vi "P4CMDSub Check for P4V.vi"(8 "error in (no error)":errorcluster) -> (0 "error out":errorcluster, 2 "visual client path":string, 5 "visual client found?":bool)   [LabVIEW 2017, in "NI_SCC_P4CMD.lvlib"]
uses:
  <vilib>/SourceControl/Providers/P4CMD/NI_SCC_P4CMD.lvlib
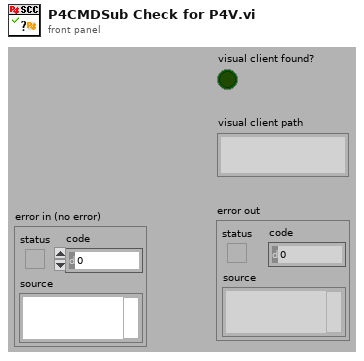
[diagram p1: front panel]
types:
  T1 = enum32{"invalid OS target", "Mac OS", "Windows 3.1", "Windows 95/NT", "Solaris 1", "Solaris 2", "HP-UX", "PowerMAX", "Linux", "Irix", "Rhapsody", "BeOS", "AIX", "OSF1", "VxWorks", "PharLap", "Carbon", "RTX", "Windows x64", "Linux x64", "Mac OS X x64"}
  T2 = enum32{"KEY_QUERY_VALUE", "KEY_SET_VALUE", "KEY_CREATE_SUB_KEY", "KEY_ENUMERATE_SUB_KEYS", "KEY_NOTIFY", "KEY_CREATE_LINK", "KEY_READ", "KEY_WRITE", "KEY_ALL_ACCESS", "KEY_READ | KEY_WRITE"}
  T3 = enum32{"HKEY_CLASSES_ROOT", "HKEY_CURRENT_USER", "HKEY_LOCAL_MACHINE", "HKEY_USERS", "HKEY_PERFORMANCE_DATA", "HKEY_CURRENT_CONFIG", "HKEY_DYN_DATA"}
  T4 = typedef "Registry refnum.ctl" = refnum<k1>
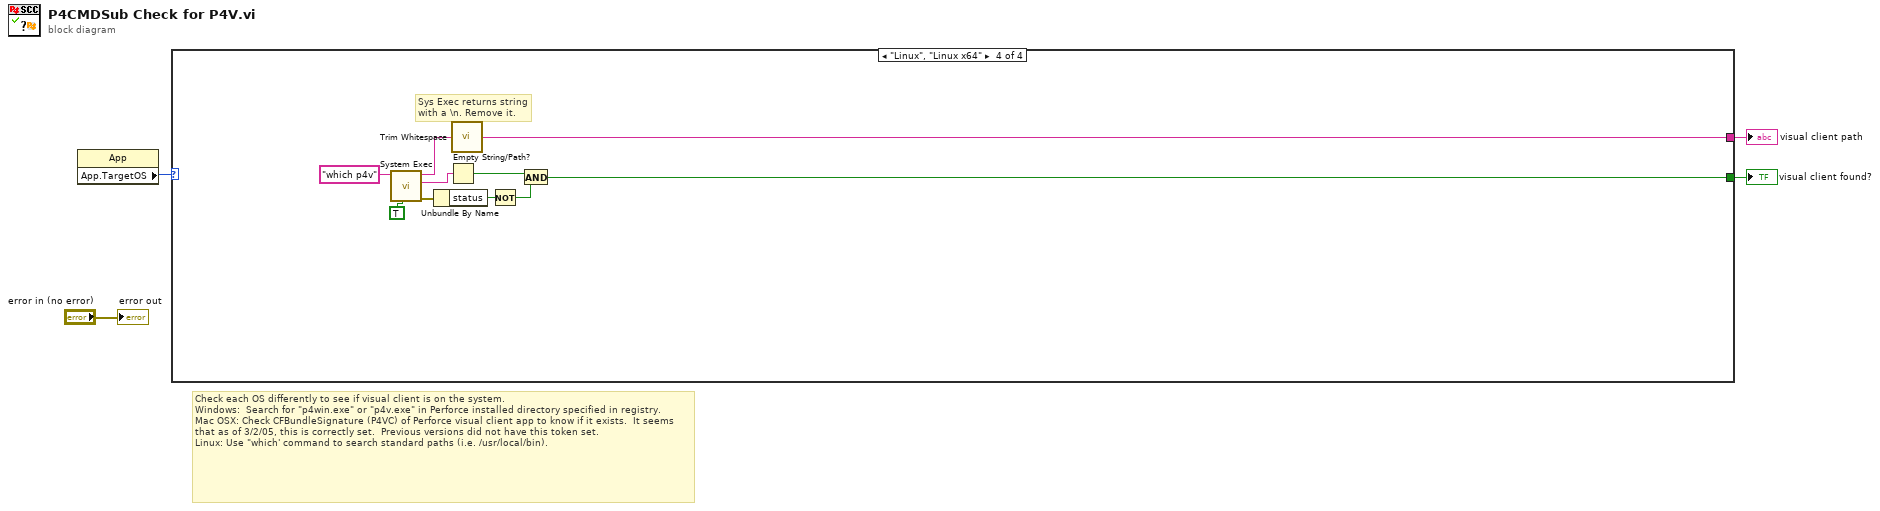
[diagram p0: block diagram]
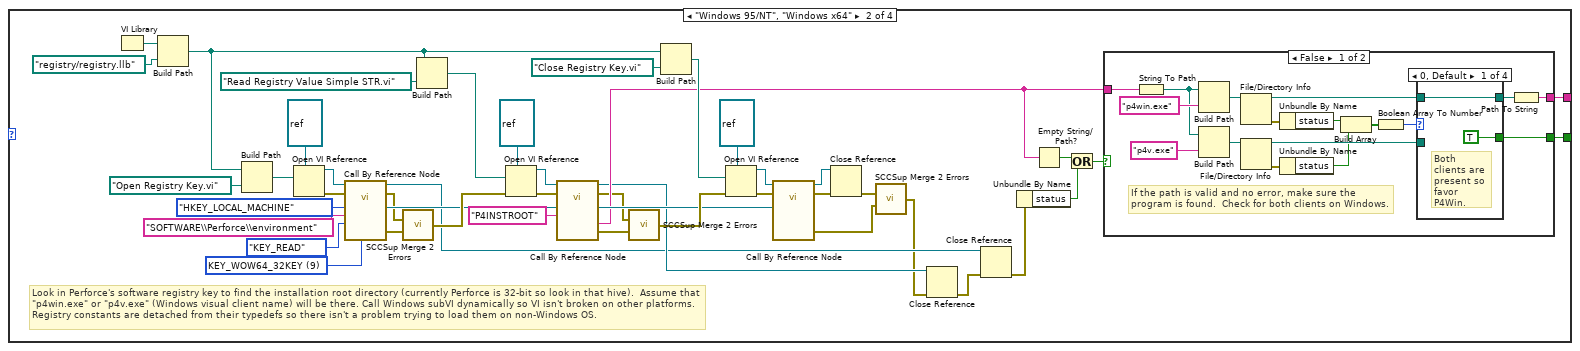
[diagram p3: hidden frame]
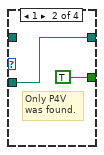
[diagram p4: hidden frame]
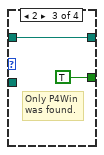
[diagram p5: hidden frame]
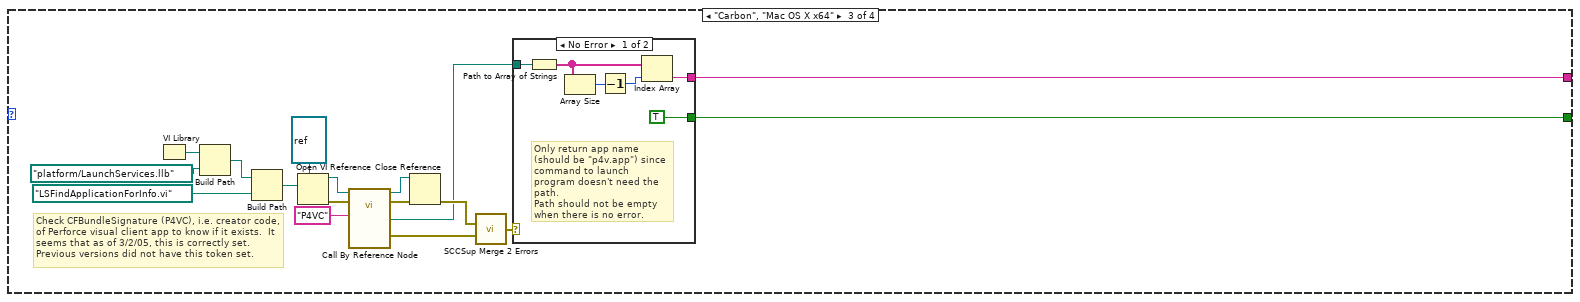
[diagram p8: hidden frame]
diagram:
  # "Check each OS differently to see if visual client is on the system. \nWindows:  Search for \"p4win.exe\" or \"p4v.exe\" in Perforce installed directory specified in registry.\nMac OSX: Check CFBundleSignature (P4VC) of Perforce visual client app to know if it exists.  It seems that as of 3/2/05, this is correctly set.  Previous versions did not have this token set.\nLinux: Use \"which' command to search standard paths (i.e. /usr/local/bin)."
  n1 = property on="Property Node" class="App"() -> ("App.TargetOS"=w3:T1)  [unwired: 2 in, 2 out]
  n2 = case shown="\"Linux\", \"Linux x64\"" w3 {
    tunnel: [_ w41 w90 w98] -> w2
    tunnel: [_ w42 w89 w97] -> w1
    frame Default {
      # "For all OS's not supporting, assume not found."
    }
    frame "Windows 95/NT", "Windows x64" {
      w5 = u16 9 items=["Default"=0, "KEY_WOW64_64KEY"=8, "KEY_WOW64_32KEY"=9] ("registry view")
      # "Look in Perforce's software registry key to find the installation root directory (currently Perforce is 32-bit so look in that hive).  Assume that \"p4win.exe\" or \"p4v.exe\" (Windows visual client name) will be there. Call Windows subVI dynamically so VI isn't broken on other platforms.  \nRegistry constants are detached from their typedefs so there isn't a problem trying to load them on non-Windows OS."
      n3 = VI Library() -> (path=w14:path)
      n4 = Build Path(base path=w14, name or relative path=path "registry/registry.llb" ("stripped path")) -> (appended path=w17:path)
      n5 = Build Path(base path=w17, name or relative path=path "Open Registry Key.vi" ("stripped path")) -> (appended path=w45:path)
      n6 = Open VI Reference(type specifier VI Refnum (for type only)=refnum<vi> refnum, vi path=w45) -> (vi reference=w47:refnum<vi>, error out=w46:errorcluster)  [unwired: 1 in, 3 out]
      n7 = call-by-ref "Call By Reference Node"(reference=w47, error in=w46, "registry view"=w5, "security access mask (KEY_READ | KEY_WRITE)"=T2."KEY_READ", "subkey"="SOFTWARE\\Perforce\\environment", "root key (HKEY_LOCAL_MACHINE)"=T3."HKEY_LOCAL_MACHINE") -> (reference out=w8:refnum<vi>, error out=w12:errorcluster, 0:"error out"=w44:errorcluster, "refnum out"=w16:T4)  [unwired: 6 in]
      n8 = call <vilib>:"SCCSup Merge 2 Errors.vi"("Error IO 1"=w12, "Error IO 2"=w44) -> ("Error IO out"=w24:errorcluster)  [unwired: 13 out]
      n9 = Build Path(base path=w17, name or relative path=path "Read Registry Value Simple STR.vi" ("stripped path")) -> (appended path=w20:path)
      n10 = Open VI Reference(type specifier VI Refnum (for type only)=refnum<vi> refnum, vi path=w20, error in (no error)=w24) -> (vi reference=w33:refnum<vi>, error out=w34:errorcluster)  [unwired: 3 out]
      n11 = call-by-ref "Call By Reference Node"(reference=w33, error in=w34, "value"="P4INSTROOT" ("subkey"), "refnum"=w16) -> (reference out=w10:refnum<vi>, error out=w11:errorcluster, 0:"error out"=w35:errorcluster, "String/Binary data"=w13:string, "refnum out"=w15:T4)  [unwired: 4 in, 1 out]
      n12 = call <vilib>:"SCCSup Merge 2 Errors.vi"("Error IO 1"=w11, "Error IO 2"=w35) -> ("Error IO out"=w21:errorcluster)  [unwired: 13 out]
      n13 = Build Path(base path=w17, name or relative path=path "Close Registry Key.vi" ("stripped path")) -> (appended path=w19:path)
      n14 = Open VI Reference(type specifier VI Refnum (for type only)=refnum<vi> refnum, vi path=w19, error in (no error)=w21) -> (vi reference=w28:refnum<vi>, error out=w27:errorcluster)  [unwired: 3 out]
      n15 = call-by-ref "Call By Reference Node"(reference=w28, error in=w27, "refnum"=w15) -> (reference out=w31:refnum<vi>, error out=w30:errorcluster, 0:"error out"=w26:errorcluster)  [unwired: 6 in]
      n16 = Close Reference(reference=w31, error in (no error)=w30) -> (error out=w25:errorcluster)
      n17 = call <vilib>:"SCCSup Merge 2 Errors.vi"("Error IO 1"=w25, "Error IO 2"=w26) -> ("Error IO out"=w7:errorcluster)  [unwired: 13 out]
      n18 = Close Reference(reference=w10, error in (no error)=w7) -> (error out=w9:errorcluster)
      n19 = Close Reference(reference=w8, error in (no error)=w9) -> (error out=w6:errorcluster)
      n20 = Unbundle By Name(w6) -> ("status"=w50:bool)
      n21 = Empty String/Path?(string/path=w13) -> (empty?=w49:bool)
      n22 = Or(x=w49, y=w50) -> (x .or. y?=w43:bool)
      n23 = case shown="False" w43 {
        tunnel: [w59 _] -> w42
        tunnel: [w67 _] -> w41
        tunnel: w13 -> [w65 _]
        frame False {
          # "If the path is valid and no error, make sure the program is found.  Check for both clients on Windows."
          n24 = String To Path(string=w65) -> (path=w62:path)
          n25 = Build Path(base path=w62, name or relative path="p4win.exe" ("subkey")) -> (appended path=w64:path)
          n26 = Build Path(base path=w62, name or relative path="p4v.exe" ("subkey")) -> (appended path=w58:path)
          n27 = File/Directory Info(path=w64) -> (path out=w61:path, error out=w57:errorcluster)  [unwired: 1 in, 5 out]
          n28 = File/Directory Info(path=w58) -> (path out=w55:path, error out=w56:errorcluster)  [unwired: 1 in, 5 out]
          n29 = Unbundle By Name(w57) -> ("status"=w54:bool)
          n30 = Unbundle By Name(w56) -> ("status"=w53:bool)
          n31 = Build Array(w54, w53) -> (w52:bool[])
          n32 = Boolean Array To Number(Boolean array=w52) -> (number=w51:u32)
          n33 = case shown="0, Default" w51 {
            tunnel: w61 -> [w68 _ w72 _]
            tunnel: [w68 w70 w72 _] -> w60
            tunnel: [TRUE TRUE TRUE _] -> w67
            tunnel: w55 -> [_ w70 _ _]
            frame 0, Default {
              # "Both clients are present so favor P4Win."
            }
            frame 1 {
              # "Only P4V was found."
            }
            frame 2 {
              # "Only P4Win was found."
            }
            frame 3 {
              # "Neither clients were found."
            }
          }
          n34 = Path To String(path=w60) -> (string=w59:string)
        }
        frame True {
          # "Path is empty or an error occurred so say client was not found."
        }
      }
    }
    frame "Carbon", "Mac OS X x64" {
      # "Check CFBundleSignature (P4VC), i.e. creator code, of Perforce visual client app to know if it exists.  It seems that as of 3/2/05, this is correctly set.  Previous versions did not have this token set."
      n35 = VI Library() -> (path=w85:path)
      n36 = Build Path(base path=w85, name or relative path=path "platform/LaunchServices.llb" ("stripped path")) -> (appended path=w86:path)
      n37 = Build Path(base path=w86, name or relative path=path "LSFindApplicationForInfo.vi" ("stripped path")) -> (appended path=w80:path)
      n38 = Open VI Reference(type specifier VI Refnum (for type only)=refnum<vi> refnum, vi path=w80) -> (vi reference=w82:refnum<vi>, error out=w81:errorcluster)  [unwired: 1 in, 3 out]
      n39 = call-by-ref "Call By Reference Node"(reference=w82, error in=w81, "creator"="P4VC") -> (reference out=w84:refnum<vi>, error out=w83:errorcluster, 0:"error out"=w76:errorcluster, "application path"=w74:path)  [unwired: 3 in]
      n40 = Close Reference(reference=w84, error in (no error)=w83) -> (error out=w77:errorcluster)
      n41 = call <vilib>:"SCCSup Merge 2 Errors.vi"("Error IO 1"=w77, "Error IO 2"=w76) -> ("Error IO out"=w75:errorcluster)  [unwired: 13 out]
      n42 = case shown="No Error" w75 {
        tunnel: [TRUE _] -> w90
        tunnel: [w91 _] -> w89
        tunnel: w74 -> [w95 _]
        frame No Error {
          # "Only return app name (should be \"p4v.app\") since command to launch program doesn't need the path.  \nPath should not be empty when there is no error."
          n43 = Path to Array of Strings(0:w95) -> (2:w93:string[])  [unwired: 1 out]
          n44 = Array Size(array=w93) -> (size(s)=w94:i32)
          n45 = Decrement(x=w94) -> (x-1=w92:i32)
          n46 = Index Array(array=w93, index=w92) -> (element=w91:string)
        }
        frame Error {
        }
      }
    }
    frame "Linux", "Linux x64" {
      # "Sys Exec returns string with a \\n. Remove it."
      n47 = call <vilib>:"System Exec.vi"("run minimized? (F)"=TRUE, "command line"="which p4v") -> ("error out"=w106:errorcluster, "standard error"=w101:string, "standard output"=w103:string)  [unwired: 4 in, 3 out]
      n48 = Unbundle By Name(w106) -> ("status"=w102:bool)
      n49 = Empty String/Path?(string/path=w101) -> (empty?=w99:bool)
      n50 = call <vilib>:"Trim Whitespace.vi"("string"=w103) -> ("trimmed string"=w97:string)  [unwired: 1 in]
      n51 = Not(x=w102) -> (.not. x?=w100:bool)
      n52 = And(x=w99, y=w100) -> (x .and. y?=w98:bool)
    }
  }
  "visual client found?" <- w2
  "visual client path" <- w1
  "error out" <- "error in (no error)"
